vi "load_dictionary.vi"   [LabVIEW 2015, in "lv-unit-conversion.lvlib"]
doc: "load_dictionary is a polymorphic VI that can be used to generate a unit dictionary using an xml or json file."
uses:
  lv-unit-conversion.lvlib
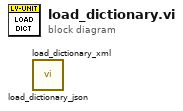
[diagram p0: block diagram]
diagram:
  n1 = call "load_dictionary_json.vi"() -> ()  [unwired: 10 in, 2 out]
  n2 = call "load_dictionary_xml.vi"() -> ()  [unwired: 10 in, 2 out]
